vi "Write Driver Setting Mappings.vi"(8 "error in (no error)":errorcluster, 10 "Driver Setting Mappings":T1[](array[typedef]), 11 "Driver in":refnum<class "Driver.lvclass">) -> (0 "error out":errorcluster, 3 "Driver out":refnum<class "Driver.lvclass">)   [LabVIEW 2023, in "HAF.lvlib" / "Driver.lvclass"]
doc: "Stores a new array of Driver Setting mappings."
uses:
  Driver.lvclass
  Driver.lvclass/Driver.ctl
  Setting Map Structure.ctl
  HAF.lvlib
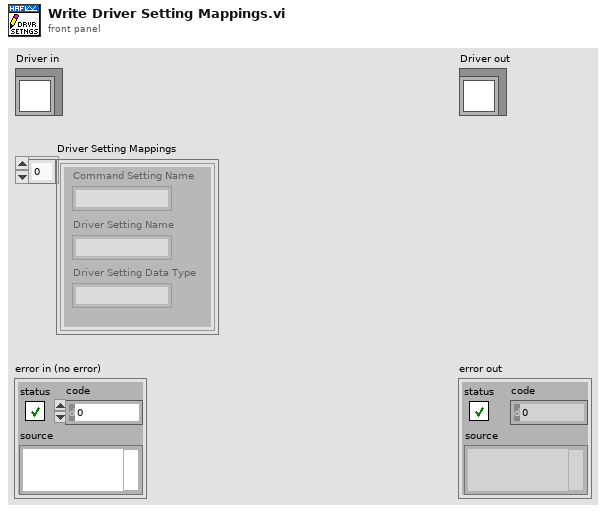
[diagram p1: front panel]
types:
  T1 = typedef "HAF.lvlib/Setting Map Structure.ctl" = cluster{"Command Setting Name":string, "Driver Setting Name":string, "Driver Setting Data Type":string}
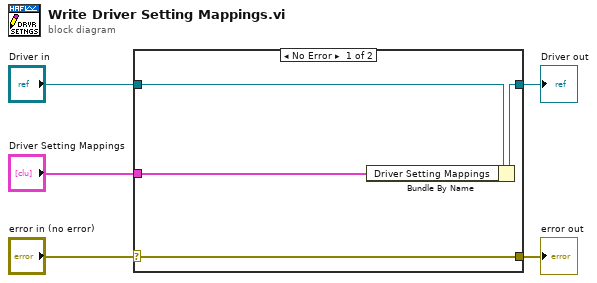
[diagram p0: block diagram]
diagram:
  n1 = case shown="No Error" "error in (no error)" {
    selector: "error in (no error)" -> [w9 w10]
    tunnel: [w9 w10] -> w4
    tunnel: [w7 w11] -> w2
    tunnel: "Driver in" -> [w8 w11]
    tunnel: "Driver Setting Mappings" -> [w6 _]
    frame No Error {
      n2 = Bundle By Name(cluster=w8, "Driver Setting Mappings"=w6) -> (w7:refnum<class "Driver.lvclass">)
    }
    frame Error {
    }
  }
  "error out" <- w4
  "Driver out" <- w2
